vi "PID_change_cte.vi"(8 "PID gains":T1, 11 "PID_Bitron in":refnum<class "PID_Bitron.lvclass">) -> (3 "PID_Bitron out":refnum<class "PID_Bitron.lvclass">)   [LabVIEW 2022 SP3, in "PID_Bitron.lvclass"]
uses:
  PID_Bitron.lvclass
  PID_Bitron.lvclass/PID_Bitron.ctl
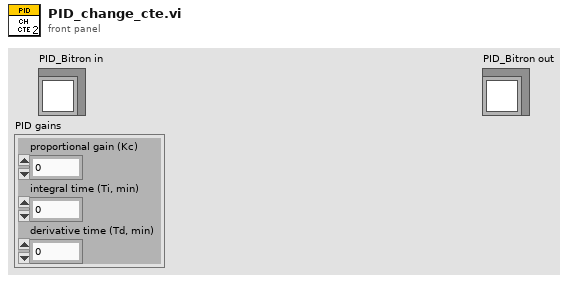
[diagram p1: front panel]
types:
  T1 = cluster{"proportional gain (Kc)":dbl, "integral time (Ti, min)":dbl, "derivative time (Td, min)":dbl}
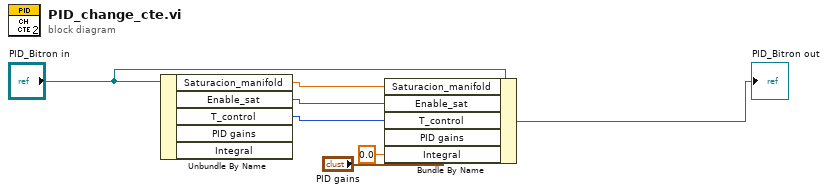
[diagram p0: block diagram]
diagram:
  n1 = Unbundle By Name("PID_Bitron in") -> ("Saturacion_manifold"=w4:dbl, "Enable_sat"=w5:bool, "T_control"=w6:enum16{"Manifold", "Bobina"})  [unwired: 2 out]
  n2 = Bundle By Name(cluster="PID_Bitron in", "Saturacion_manifold"=w4, "Enable_sat"=w5, "T_control"=w6, "PID gains"="PID gains", "Integral"=0.0) -> (→"PID_Bitron out":refnum<class "PID_Bitron.lvclass">)
